vi "GE 5565PIORC.PIO.Window.Set Local Base Address.vi"(8 "error in (no error)":errorcluster, 10 "local base address":u32 format="%.0x", 11 "GE 5565PIORC in":refnum<class "GE 5565PIORC.lvclass">) -> (0 "error out":errorcluster, 3 "GE 5565PIORC out":refnum<class "GE 5565PIORC.lvclass">)   [LabVIEW 2016, in "GE 5565PIORC.lvclass"]
doc: "Sets the <B>local base address</B> to use for windowed PIO reads and writes. Any offset will be used relative to the local base address to get an absolute address in reflective memory."
uses:
  GE 5565PIORC.lvclass
  GE 5565PIORC.lvclass/GE 5565PIORC.ctl
  Properties/Registers/GE 5565PIORC.Registers.Local Configuration.Read.vi
  Properties/Registers/GE 5565PIORC.Registers.Local Configuration.Read (U32).vi
  Properties/Registers/GE 5565PIORC.Registers.Local Configuration.Write.vi
  Properties/Registers/GE 5565PIORC.Registers.Local Configuration.Write (U32).vi
  Properties/Registers/GE 5565PIORC.Registers.Read.vi
  Properties/Registers/GE 5565PIORC.Registers.Read (U32).vi
  Properties/Registers/GE 5565PIORC.Registers.Write.vi
  Properties/Registers/GE 5565PIORC.Registers.Write (U32).vi
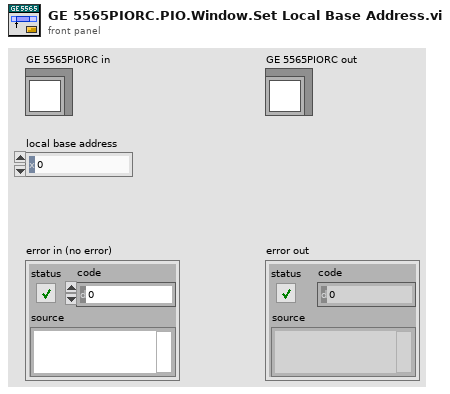
[diagram p1: front panel]
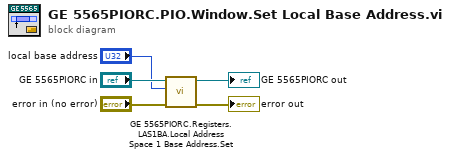
[diagram p0: block diagram]
diagram:
  n1 = call "GE 5565PIORC.Registers.LAS1BA.Local Address Space 1 Base Address.Set.vi"("error in (no error)"="error in (no error)", "Local Address Space 1 Base Address"="local base address", "GE 5565PIORC in"="GE 5565PIORC in") -> ("error out"=→"error out":errorcluster, "GE 5565PIORC out"=→"GE 5565PIORC out":refnum<class "GE 5565PIORC.lvclass">)  [unwired: 7 in]
